vi "Special Mouse Coordinates.vi"(0 "Mouse Click Coordinates":T2) -> (1 "Special Case (Last, Selected, All)":bool, 2 "Special Coordinates Case":T1)   [LabVIEW 2021, in "Graphs.lvlib"]
uses:
  Graphs.lvlib
  <vilib>/Utility/miscctls.llb/LVPoint32TypeDef.ctl
  Graph Legend Special Coordinates.ctl
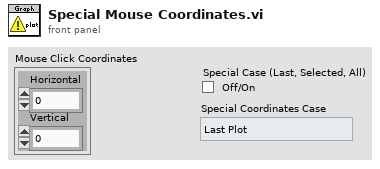
[diagram p1: front panel]
types:
  T1 = typedef "Graphs.lvlib/Graph Legend Special Coordinates.ctl" = enum16{"Last Plot", "Selected Plots", "All Plots"}
  T2 = typedef "LVPoint32TypeDef.ctl" = cluster{"Horizontal":i32, "Vertical":i32}
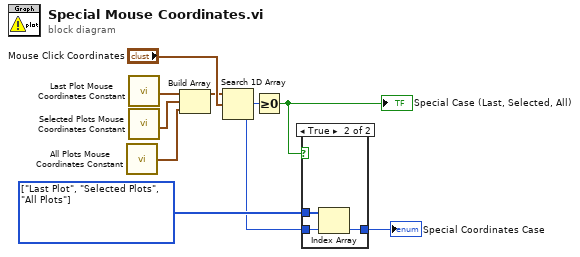
[diagram p0: block diagram]
diagram:
  w5 = T1[] [enum."Last Plot", enum."Selected Plots", enum."All Plots"] items=["Last Plot", "Selected Plots", "All Plots"] ("Array")
  n1 = call "All Plots Mouse Coordinates Constant.vi"() -> ("Selected Plots Mouse Coordinates Equivalent"=w1:T2)
  n2 = call "Last Plot Mouse Coordinates Constant.vi"() -> ("Selected Plots Mouse Coordinates Equivalent"=w7:T2)
  n3 = call "Selected Plots Mouse Coordinates Constant.vi"() -> ("Selected Plots Mouse Coordinates Equivalent"=w2:T2)
  n4 = Build Array(w7, w2, w1) -> (w8:T2[])
  n5 = Search 1D Array(1D array=w8, element="Mouse Click Coordinates") -> (index of element=w4:i32)  [unwired: 1 in]
  n6 = Greater Or Equal To 0?(x=w4) -> (x >= 0?=w6:bool)
  "Special Case (Last, Selected, All)" <- w6
  n7 = case shown="True" w6 {
    tunnel: w5 -> [_ w12]
    tunnel: w4 -> [_ w11]
    tunnel: [_ w10] -> w3
    frame False {
    }
    frame True {
      n8 = Index Array(array=w12, index=w11) -> (element=w10:T1)
    }
  }
  "Special Coordinates Case" <- w3
